vi "2D.vi"() -> ()   [LabVIEW 2023]
uses:
  <vilib>/Utility/file.llb/Read Delimited Spreadsheet (string).vi
panel:
  out "Array 3":i32[](array[numeric])
  out "Array 2":i32[][](array[numeric])
  out "Array":i32[][](array[numeric])
  out "Last Result":i32[][][](array[numeric])
  out "?":i32[][][](array[numeric])
  # "All Results"
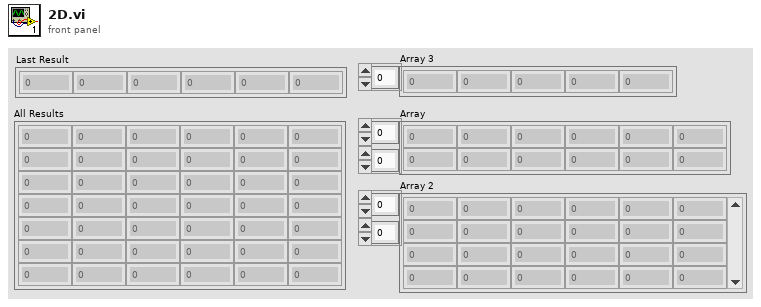
[diagram p1: front panel]
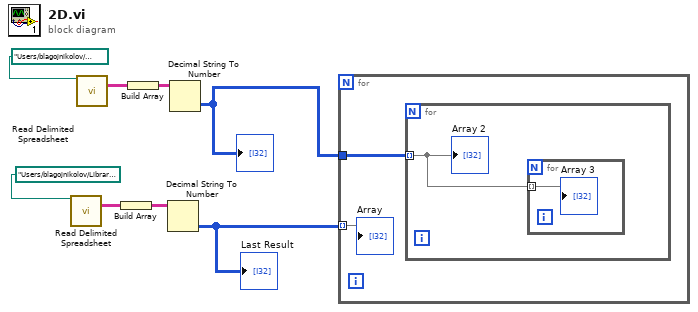
[diagram p0: block diagram]
diagram:
  n1 = call-poly <vilib>:"Read Delimited Spreadsheet.vi"("file path (dialog if empty)"=path "/Users/blagojnikolov/Library/Mobile Documents/com~apple~CloudDocs/TOTO/LastResult.txt") -> ("all rows"=w6:string[][])  [unwired: 9 in, 5 out]
  n2 = call-poly <vilib>:"Read Delimited Spreadsheet.vi"("file path (dialog if empty)"=path "/Users/blagojnikolov/Desktop/@tmp/archive1.txt") -> ("all rows"=w8:string[][])  [unwired: 9 in, 5 out]
  n3 = Build Array(w6) -> (w5:string[][][])
  n4 = Build Array(w8) -> (w3:string[][][])
  n5 = Decimal String To Number(string=w5) -> (number=w1:i32[][][])  [unwired: 2 in, 1 out]
  "Last Result" <- w1
  n6 = Decimal String To Number(string=w3) -> (number=w2:i32[][][])  [unwired: 2 in, 1 out]
  "?" <- w2
  n7 = for {
    tunnel: w2 -> [w10]
    tunnel: w1 -> [w9] mode=indexing
    n8 = for {
      tunnel: w10 -> [w11] mode=indexing
      n9 = for {
        tunnel: w11 -> [w12] mode=indexing
        "Array 3" <- w12
      }
      "Array 2" <- w11
    }
    "Array" <- w9
  }
